vi "emi_Merge Error Simple.vi"(4 "merge":errorcluster, 5 "error in":errorcluster) -> (1 "error out":errorcluster)   [LabVIEW 2010]
doc: "DEPRECATED. Replaced in 2010 by buildt in funcion. Can be used to reduce rrom\n\nError In == Error. Merge == Error. Error Out = Error In\nError In == Error. Merge != Error. Error Out = Error In\nError In != Error. Merge == Error. Error Out = Merge\nError In != Error. Merge != Error. Error Out = Error In\n\nReentrant subroutine for performance."
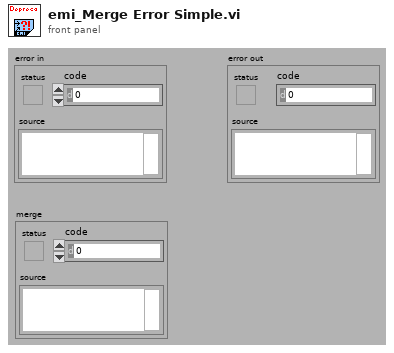
[diagram p1: front panel]
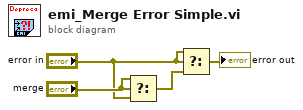
[diagram p0: block diagram]
diagram:
  n1 = Select(t="merge", s="merge", f="error in") -> (s? t:f=w3:errorcluster)
  n2 = Select(t="error in", s="error in", f=w3) -> (s? t:f=→"error out":errorcluster)
